vi "曲线属性.vi"(11 "曲线":cluster{"测试数据":dbl[], "测试数据":dbl[]}[](array[cluster])) -> (3 "曲线属性":T1[](array[typedef]))   [LabVIEW 2021]
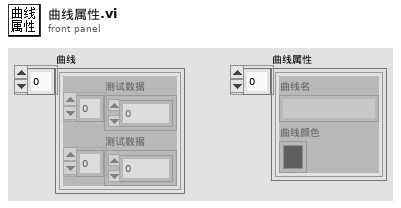
[diagram p1: front panel]
types:
  T1 = typedef "曲线属性.ctl" = cluster{"曲线名":string, "曲线颜色":u32}
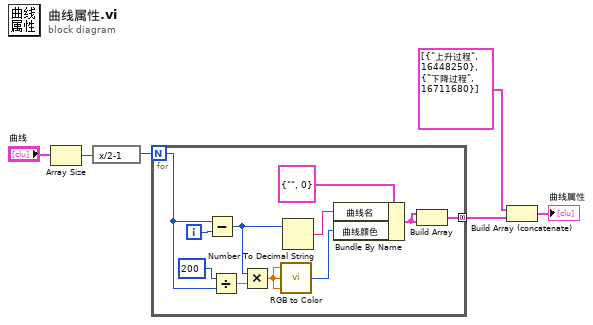
[diagram p0: block diagram]
diagram:
  n1 = Array Size(array="曲线") -> (size(s)=w5:i32)
  n2 = expression code="x/2-1"(w5) -> (w6:i32)
  n3 = for {
    N: w6 -> [w16]
    tunnel: [w10] -> w2 mode=concatenating
    i -> [w15]
    n4 = Subtract(x=w16, y=w15) -> (x-y=w7:i32)
    n5 = Divide(x=200, y=w16) -> (x/y=w8:dbl)
    n6 = Multiply(x=w7, y=w8) -> (x*y=w14:dbl)
    n7 = call <vilib>:"RGB to Color.vi"("B"=w14, "G"=w14, "R"=w14) -> ("Color"=w12:u32)
    n8 = Number To Decimal String(number=w7) -> (decimal integer string=w9:string)  [unwired: 1 in]
    n9 = Bundle By Name(cluster=T1 {"曲线名"="", "曲线颜色"=0} ("曲线属性"), "曲线名"=w9, "曲线颜色"=w12) -> (w11:T1)
    n10 = Build Array(w11, w11) -> (w10:T1[])
  }
  n11 = Build Array (concatenate)(T1[] [{"曲线名"="上升过程", "曲线颜色"=16448250}, {"曲线名"="下降过程", "曲线颜色"=16711680}], w2) -> (→"曲线属性":T1[])
